vi "SeCrTS-DD NS Receiver Pump.vi"(8 "error in":errorcluster) -> ()   [LabVIEW 2022 SP3]
uses:
  Control/SeCrTS-Notifier Ref.ctl
  Globals/SeCrTS-DD globals.vi
  <resource>/objmgr/ni.dex.rc
panel:
  out "x":u32
  out "error out":errorcluster
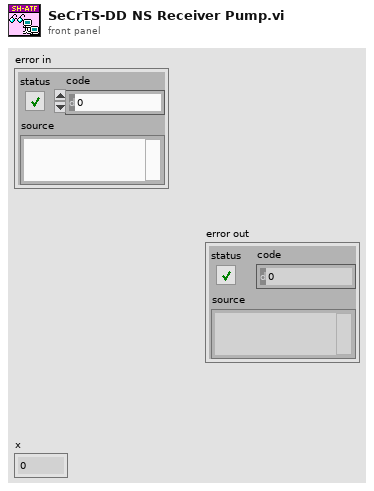
[diagram p1: front panel]
types:
  T1 = typedef "SeCrTS-Notifier Ref.ctl" = cluster{"Pump":refnum<notifier>, "Storage":refnum<notifier>}
  T2 = cluster{"In Progress":bool, "reader url":refnum<k21>, "DI P\nDI S":refnum<queue>[], "Analog Queue":refnum<queue>[], "NOT DIS Out":T1}
  T3 = enum16{"Initialize", "Wait for connection", "Send data", "Exit", "Receive Data"}
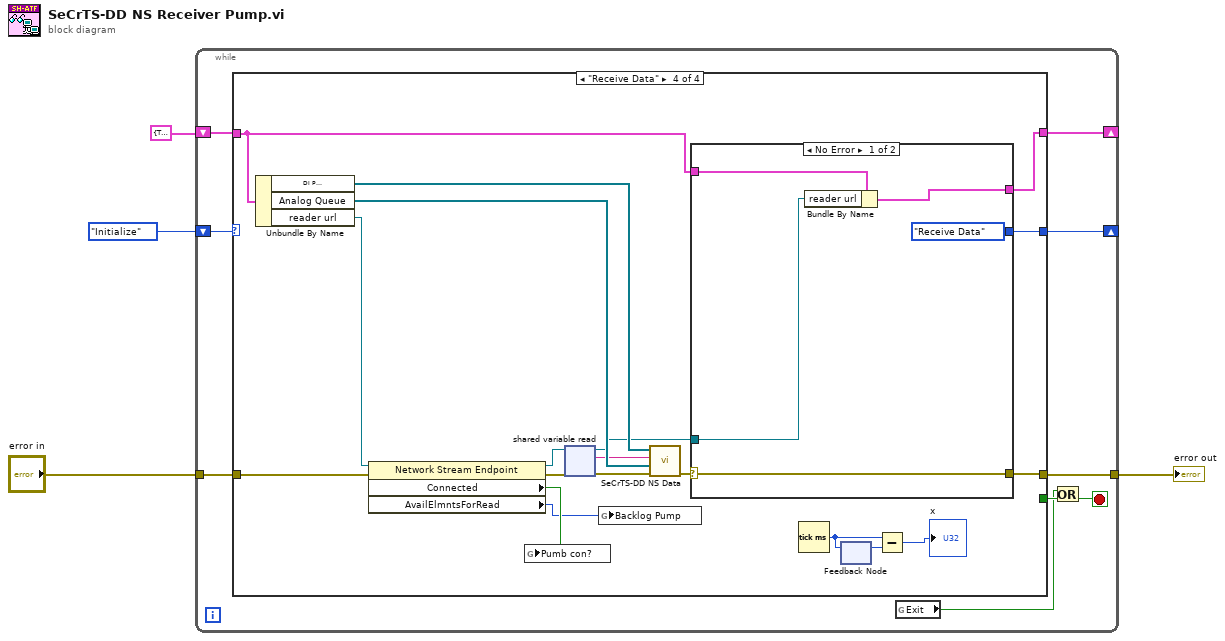
[diagram p0: block diagram]
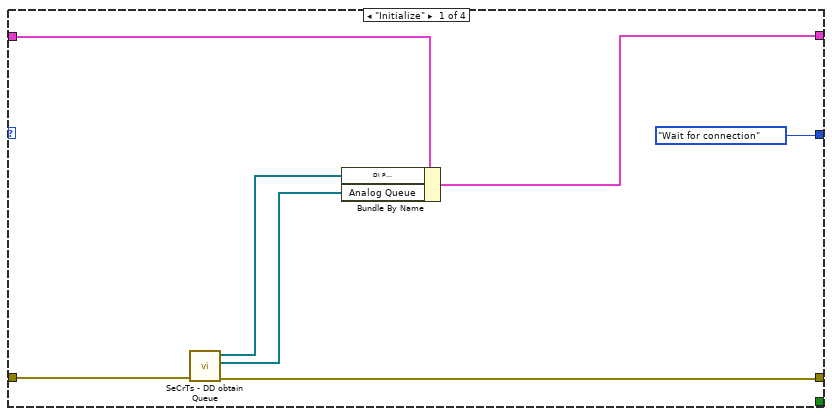
[diagram p2: hidden frame]
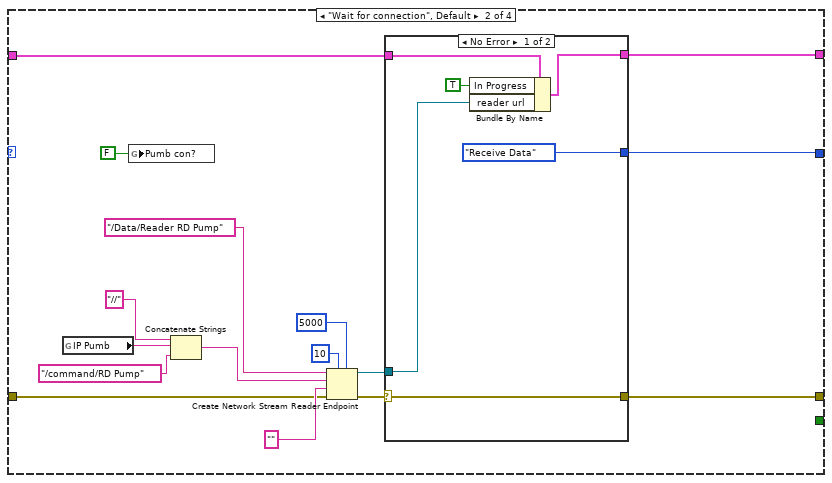
[diagram p3: hidden frame]
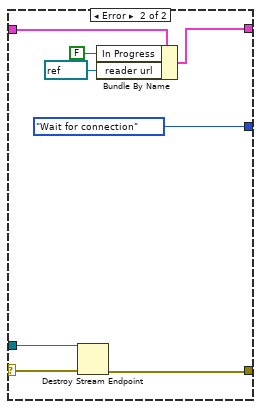
[diagram p4: hidden frame]
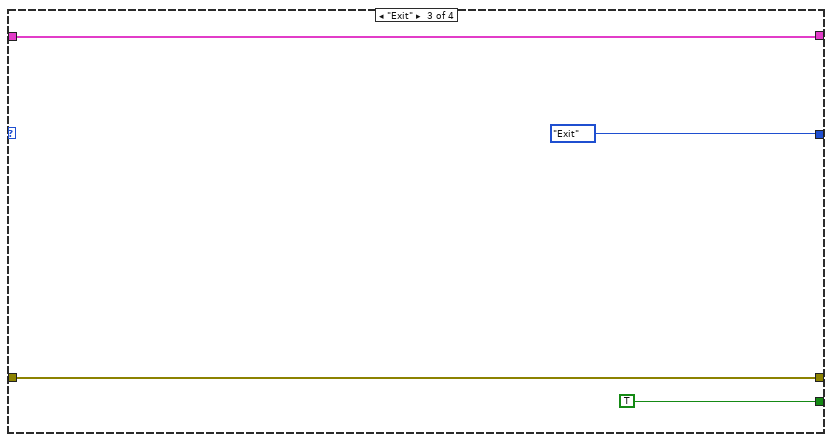
[diagram p5: hidden frame]
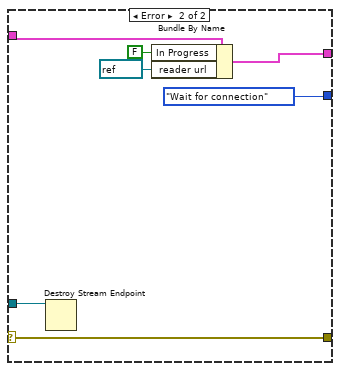
[diagram p6: hidden frame]
diagram:
  n1 = while {
    shift-right: [w11] -> _
    shift-left: T3."Initialize" -> [w13]
    shift-right: [w9] -> _
    shift-left: T2 {"In Progress"=TRUE, "reader url"="", "DI P\nDI S"=[], "Analog Queue"=[], "NOT DIS Out"={"Pump"=refnum, "Storage"=refnum}} -> [w10]
    tunnel: "error in" -> [w6]
    tunnel: [w5] -> w1
    stop <- w8 stop-if-true
    n2 = case shown="\"Receive Data\"" w13 {
      tunnel: [_ _ TRUE _] -> w12
      tunnel: [T3."Wait for connection" w33 T3."Exit" w60] -> w11
      tunnel: w10 -> [w17 w36 w53 w56]
      tunnel: [w16 w35 w53 w55] -> w9
      tunnel: [w18 w34 w51 w58] -> w5
      tunnel: w6 -> [w19 w23 w51 w66]
      frame "Initialize" {
        n3 = call "SeCrTs - DD obtain Queue.vi"("error in"=w19) -> ("error out"=w18:errorcluster, "AI_V_Data P\nAI_C_Data P\nAO_Data P\nDO_Data P\nACC_Data P\nTC Data P\nDrive_A_C \nDrive_A_D\nAI_C_Data S\nDO_Data S\nAI_V_Rms_P"=w14:refnum<queue>[], "DI P\nDI S"=w15:refnum<queue>[])  [unwired: 8 in]
        n4 = Bundle By Name(cluster=w17, "DI P\nDI S"=w15, "Analog Queue"=w14) -> (w16:T2)
      }
      frame "Wait for connection", Default {
        n5 = global read "SeCrTS-DD globals.vi" "IP Pumb"() -> (w26:string)
        n6 = global write "SeCrTS-DD globals.vi" "Pumb con?"(FALSE ("Storage con?")) -> ()
        n7 = Concatenate Strings("//" ("string"), w26, "/command/RD Pump" ("reader url")) -> (w21:string)
        n8 = Create Network Stream Reader Endpoint(5:5000 ("timeout in ms (-1)"), 7:10 ("reader buffer size"), 8:w23, 9:"", 10:w21, 11:"/Data/Reader RD Pump") -> (0:w30:errorcluster, 3:w31:refnum<k21>)  [unwired: 1 in]
        n9 = case shown="No Error" w30 {
          selector: w30 -> [w39 w46]
          tunnel: w36 -> [w42 w50]
          tunnel: w31 -> [w37 w47]
          tunnel: [w40 w49] -> w35
          tunnel: [w39 w45] -> w34
          tunnel: [T3."Receive Data" T3."Wait for connection"] -> w33
          frame No Error {
            n10 = Bundle By Name(cluster=w42, "In Progress"=TRUE, "reader url"=w37) -> (w40:T2)
          }
          frame Error {
            n11 = Destroy Stream Endpoint(8:w46, 11:w47) -> (0:w45:errorcluster)
            n12 = Bundle By Name(cluster=w50, "In Progress"=FALSE, "reader url"=refnum<k21> refnum) -> (w49:T2)
          }
        }
      }
      frame "Exit" {
      }
      frame "Receive Data" {
        n13 = Unbundle By Name(w56) -> ("DI P\nDI S"=w64:refnum<queue>[], "Analog Queue"=w63:refnum<queue>[], "reader url"=w57:refnum<k21>)
        n14 = property class="Network Stream Endpoint"(reference=w57, error in=w66) -> (reference out=w73:refnum<k21>, error out=w72:errorcluster, "Connected"=w71:bool, "AvailElmntsForRead"=w67:i32)
        n15 = global write "SeCrTS-DD globals.vi" "Pumb con?"(w71) -> ()
        n16 = shared-variable-read(w73, w72) -> (w59:refnum<k21>, w65:errorcluster, w62:string)  [unwired: 1 in, 1 out]
        n17 = global write "SeCrTS-DD globals.vi" "Backlog Pump"(w67) -> ()
        n18 = call "SeCrTS-DD NS Data.vi"("error in"=w65, "AI_V_Data P\nAI_C_Data P\nAO_Data P\nDO_Data P\nACC_Data P\nTC Data P\nDrive_A_C \nDrive_A_D\nAI_C_Data S\nDO_Data S\nAI_V_Rms_P"=w63, "data out"=w62, "DI P\nDI S"=w64) -> ("error out"=w61:errorcluster)  [unwired: 7 in]
        n19 = case shown="No Error" w61 {
          selector: w61 -> [w78 w85]
          tunnel: [w78 w85] -> w58
          tunnel: [T3."Receive Data" T3."Wait for connection"] -> w60
          tunnel: w59 -> [w74 w83]
          tunnel: w56 -> [w75 w82]
          tunnel: [w76 w80] -> w55
          frame No Error {
            n20 = Bundle By Name(cluster=w75, "reader url"=w74) -> (w76:T2)
          }
          frame Error {
            n21 = Destroy Stream Endpoint(11:w83) -> ()  [unwired: 1 in, 1 out]
            n22 = Bundle By Name(cluster=w82, "In Progress"=FALSE, "reader url"=refnum<k21> refnum) -> (w80:T2)
          }
        }
        n23 = Tick Count (ms)() -> (millisecond timer value=w69:u32)
        n24 = feedback #1() -> (w70:u32)  [unwired: 1 in]
        n25 = feedback-in #1(w69) -> ()
        n26 = Subtract(x=w69, y=w70) -> (x-y=→"x":u32)
      }
    }
    n27 = global read "SeCrTS-DD globals.vi" "Exit"() -> (w7:bool)
    n28 = Or(x=w7, y=w12) -> (x .or. y?=w8:bool)
  }
  "error out" <- w1
